vi "Untitled 4 (SubVI).vi"(11 "RPM":dbl) -> (3 "Numeric":dbl)   [LabVIEW 2026]
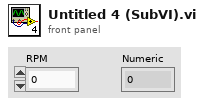
[diagram p1: front panel]
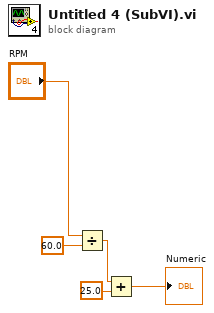
[diagram p0: block diagram]
diagram:
  n1 = Divide(x="RPM", y=60.0) -> (x/y=w3:dbl)
  n2 = Add(x=w3, y=25.0) -> (x+y=→"Numeric":dbl)
